vi "test_Add Command_Variable Duplicate Error.vi"(8 "error in (no error)":errorcluster, 11 "TestCase in":refnum<class "Instrument Addon Scripting API Messages Unit Tests.lvclass">) -> (0 "error out":errorcluster, 3 "TestCase out":refnum<class "Instrument Addon Scripting API Messages Unit Tests.lvclass">)   [LabVIEW 2019, in "Instrument Addon Scripting API Messages Unit Tests.lvclass"]
uses:
  Instrument Addon Scripting API Messages Unit Tests.lvclass
  APIs/Scripting API/TypeDefs/Command Settings.ctl
  <vilib>/NI VeriStand/Custom Device API/Custom Device Item Ref.ctl
  APIs/Scripting API/TypeDefs/Padding.ctl
  Instrument Addon Scripting API Messages Unit Tests.lvclass/Instrument Addon Scripting API Messages Unit Tests.ctl
  Addon/Addon Shared/SubVIs/Constants.vi
  <vilib>/NI/NI VeriStand Advanced SysDef API/_SubVIs/SysDef.Search.GUID.vi
  <vilib>/addons/_JKI Toolkits/VI Tester/TestCase.llb/TestCase.lvclass
  <vilib>/NI/NI VeriStand Advanced SysDef API/SysDef API/Advanced System Definition.lvlib
  Addon/Addon Shared/Instrument Addon Shared.lvlib
  <vilib>/NI VeriStand/Custom Device API/Custom Device API.lvlib
  APIs/Scripting API/Instrument Addon Scripting API.lvlib
  C:/Program Files (x86)/National Instruments/LabVIEW 2019/vi.lib/addons/_JKI Toolkits/VI Tester/TestCase.llb/TestCase.lvclass
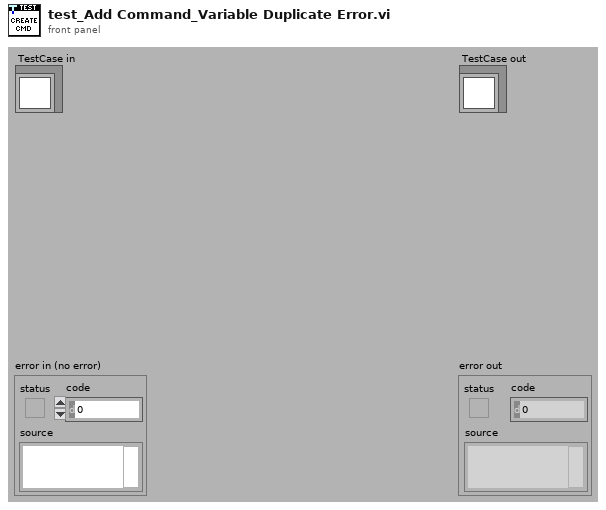
[diagram p1: front panel]
types:
  T1 = typedef "Instrument Addon Scripting API.lvlib/Command Settings.ctl" = cluster{"Command Format":string, "Linked Channels":cluster{"Variable Name":string, "Channel Ref in":T2}[], "Use Padding?":bool, "Padding":T3}
  T2 = typedef "Custom Device API.lvlib/Custom Device Item Ref.ctl" = u64
  T3 = typedef "Instrument Addon Scripting API.lvlib/Padding.ctl" = cluster{"Pad Value":u8, "Length":u32}
  T4 = typedef "Instrument Addon Scripting API.lvlib/Linked Channel.ctl" = cluster{"Variable Name":string, "Channel Refnum":T2}
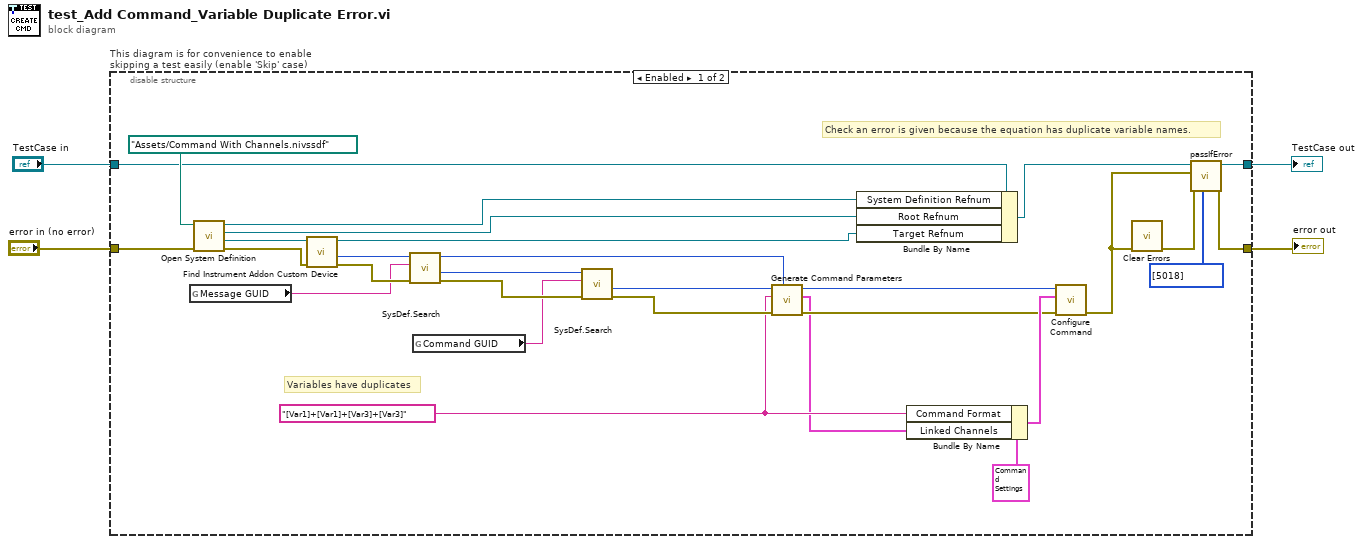
[diagram p0: block diagram]
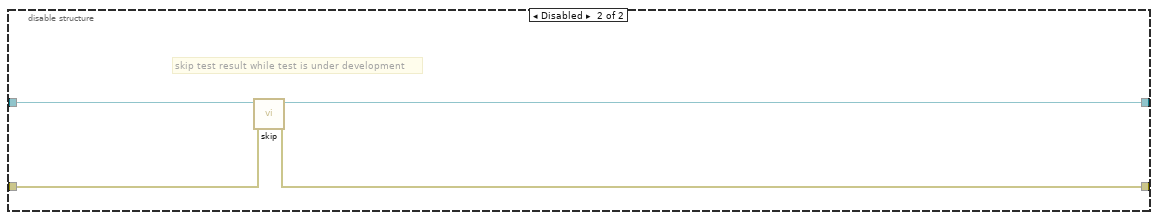
[diagram p2: hidden frame]
diagram:
  n1 = disable-structure "This diagram is for convenience to enable skipping a test easily (enable 'Skip' case)" shown="Enabled" {
    disable-tunnel: "TestCase in" -> [w21 w37]
    disable-tunnel: [w30 w35] -> w1
    disable-tunnel: [w31 w36] -> w3
    disable-tunnel: "error in (no error)" -> [w32 w34]
    frame Enabled {
      w7 = "[Var1]+[Var1]+[Var3]+[Var3]" ("Command Format")
      # "Variables have duplicates"
      # "Check an error is given because the equation has duplicate variable names."
      n2 = global read "Constants.vi" "Message GUID"() -> (w26:string)
      n3 = call "Open System Definition.vi"("error in (no error)"=w32, "System Definition File"=path "Assets/Command With Channels.nivssdf" ("SDF file")) -> ("error out"=w28:errorcluster, "Target Refnum"=w29:refnum<k24>, "Root Refnum"=w18:refnum<k24>, "System Definition Refnum"=w19:refnum<k24>)  [unwired: 6 in]
      n4 = call "Find Instrument Addon Custom Device.vi"("error in"=w28, "target in"=w29) -> ("error out"=w27:errorcluster, "NodeID"=w24:u64, "target out"=w17:refnum<k24>)  [unwired: 7 in]
      n5 = call-poly <vilib>:"SysDef.Search.vi"("error in (no error)"=w27, "GUID"=w26, "nodeID"=w24) -> ("error out"=w13:errorcluster, "Value out"=w14:u64, "nodeID out"=w5:u64)  [unwired: 5 in, 1 out]
      n6 = global read "Constants.vi" "Command GUID"() -> (w12:string)
      n7 = call-poly <vilib>:"SysDef.Search.vi"("error in (no error)"=w13, "GUID"=w12, "nodeID"=w14) -> ("error out"=w9:errorcluster, "Value out"=w11:u64)  [unwired: 5 in, 2 out]
      n8 = call "Generate Command Parameters.vi"("Instrument Addon Refnum in"=w5, "Error In"=w9, "Command String"=w7, "Command Channel in"=w11) -> ("Error Out"=w8:errorcluster, "Linked Channels"=w6:T4[], "Command Channel out"=w10:T2)  [unwired: 4 in, 1 out]
      n9 = Bundle By Name(cluster=w21, "System Definition Refnum"=w19, "Root Refnum"=w18, "Target Refnum"=w17) -> (w20:refnum<class "Instrument Addon Scripting API Messages Unit Tests.lvclass">)
      n10 = Bundle By Name(cluster=T1 {"Command Format"="[Var1]+[Var2]", "Linked Channels"=[{"Variable Name"="Var1", "Channel Ref in"=32}, {"Variable Name"="Var2", "Channel Ref in"=33}], "Use Padding?"=FALSE, "Padding"={"Pad Value"=0, "Length"=0}} ("Settings"), "Command Format"=w7, "Linked Channels"=w6) -> (w15:T1)
      n11 = call "Configure Command.vi"("error in (no error)"=w8, "settings"=w15, "command refnum in"=w10) -> ("error out"=w16:errorcluster)  [unwired: 7 in, 1 out]
      n12 = call <vilib>:"Clear Errors.vi"("error in (no error)"=w16) -> ("error out"=w22:errorcluster)  [unwired: 5 in, 1 out]
      n13 = call-dynamic "passIfError.vi"("passing error codes (default = any error code)"=i32[] [5018], "error in (no error)"=w22, "error"=w16, "TestCase in"=w20) -> ("error out"=w31:errorcluster, "TestCase out"=w30:refnum<class "Instrument Addon Scripting API Messages Unit Tests.lvclass">)  [unwired: 6 in]
    }
    frame Disabled {
      # "skip test result while test is under development"
      n14 = call <vilib>:"skip.vi"("error in (no error)"=w34, "TestCase in"=w37) -> ("error out"=w36:errorcluster, "TestCase out"=w35:refnum<class "Instrument Addon Scripting API Messages Unit Tests.lvclass">)  [unwired: 8 in]
    }
  }
  "error out" <- w3
  "TestCase out" <- w1
